vi "AprilTagFieldLayout_New2023.vi"() -> (3 "AprilTagFieldLayout":T1={"AprilTagMap"={}, "FieldLength"=0.0, "FieldWidth"=0.0, "OriginPosition "=enum."kBlueAllianceWallRightSide,", "OriginPose3d"={"Translation3d"={"X"=0.0, "Y"=0.0, "Z"=0.0}, "Rotation3d"={"Q_quaternion"={"R"=1.0, "V"=[0.0, 0.0, 0.0]}}}} {"OriginPose3d"."Translation3d"."Z" format="%14.3f"; "OriginPose3d"."Translation3d"."Y" format="%14.3f"; "OriginPose3d"."Translation3d"."X" format="%14.3f"})   [LabVIEW 2019, in "Trajectory_Library.lvlib"]
doc: "Define the FRC 2023 April Tag field layout.\n\nInputs:\n <none>\n\nOutputs:\n -- AprilTagFieldLayout -- AprilTagFieldLayout -- Data cluster containing field definition."
uses:
  Trajectory_Library.lvlib
  TypeDef/AprilTagFieldLayout.ctl
  TypeDef/AprilTag.ctl
  TypeDef/POSE3D.ctl
  TypeDef/TRANSLATION3D.ctl
  TypeDef/ROTATION3D.ctl
  TypeDef/QUATERNION.ctl
  Enum/AprilTagFieldLayoutOrignPosition_ENUM.ctl
  AprilTag_GetAll.vi
  Quaternion_Normalize.vi
  Quaternion_New_Default.vi
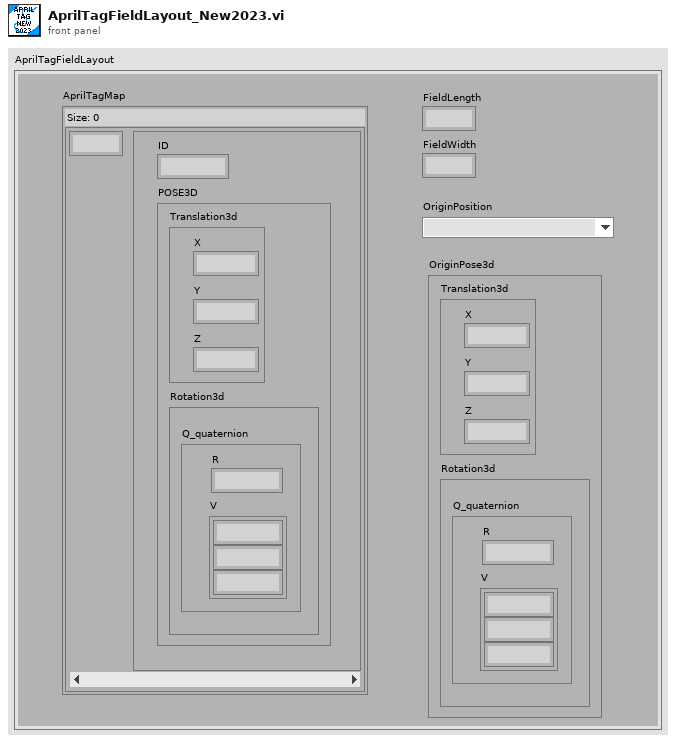
[diagram p1: front panel]
types:
  T1 = typedef "Trajectory_Library.lvlib/AprilTagFieldLayout.ctl" = cluster{"AprilTagMap":map{i32, T2}, "FieldLength":dbl, "FieldWidth":dbl, "OriginPosition ":T7, "OriginPose3d":T3}
  T2 = typedef "Trajectory_Library.lvlib/AprilTag.ctl" = cluster{"ID":i32, "POSE3D":T3}
  T3 = typedef "Trajectory_Library.lvlib/POSE3D.ctl" = cluster{"Translation3d":T4, "Rotation3d":T5}
  T4 = typedef "Trajectory_Library.lvlib/TRANSLATION3D.ctl" = cluster{"X":dbl, "Y":dbl, "Z":dbl}
  T5 = typedef "Trajectory_Library.lvlib/ROTATION3D.ctl" = cluster{"Q_quaternion":T6}
  T6 = typedef "Trajectory_Library.lvlib/QUATERNION.ctl" = cluster{"R":dbl, "V":dbl[]}
  T7 = typedef "Trajectory_Library.lvlib/AprilTagFieldLayoutOrignPosition_ENUM.ctl" = enum16{"kBlueAllianceWallRightSide,", "kRedAllianceWallRightSide,"}
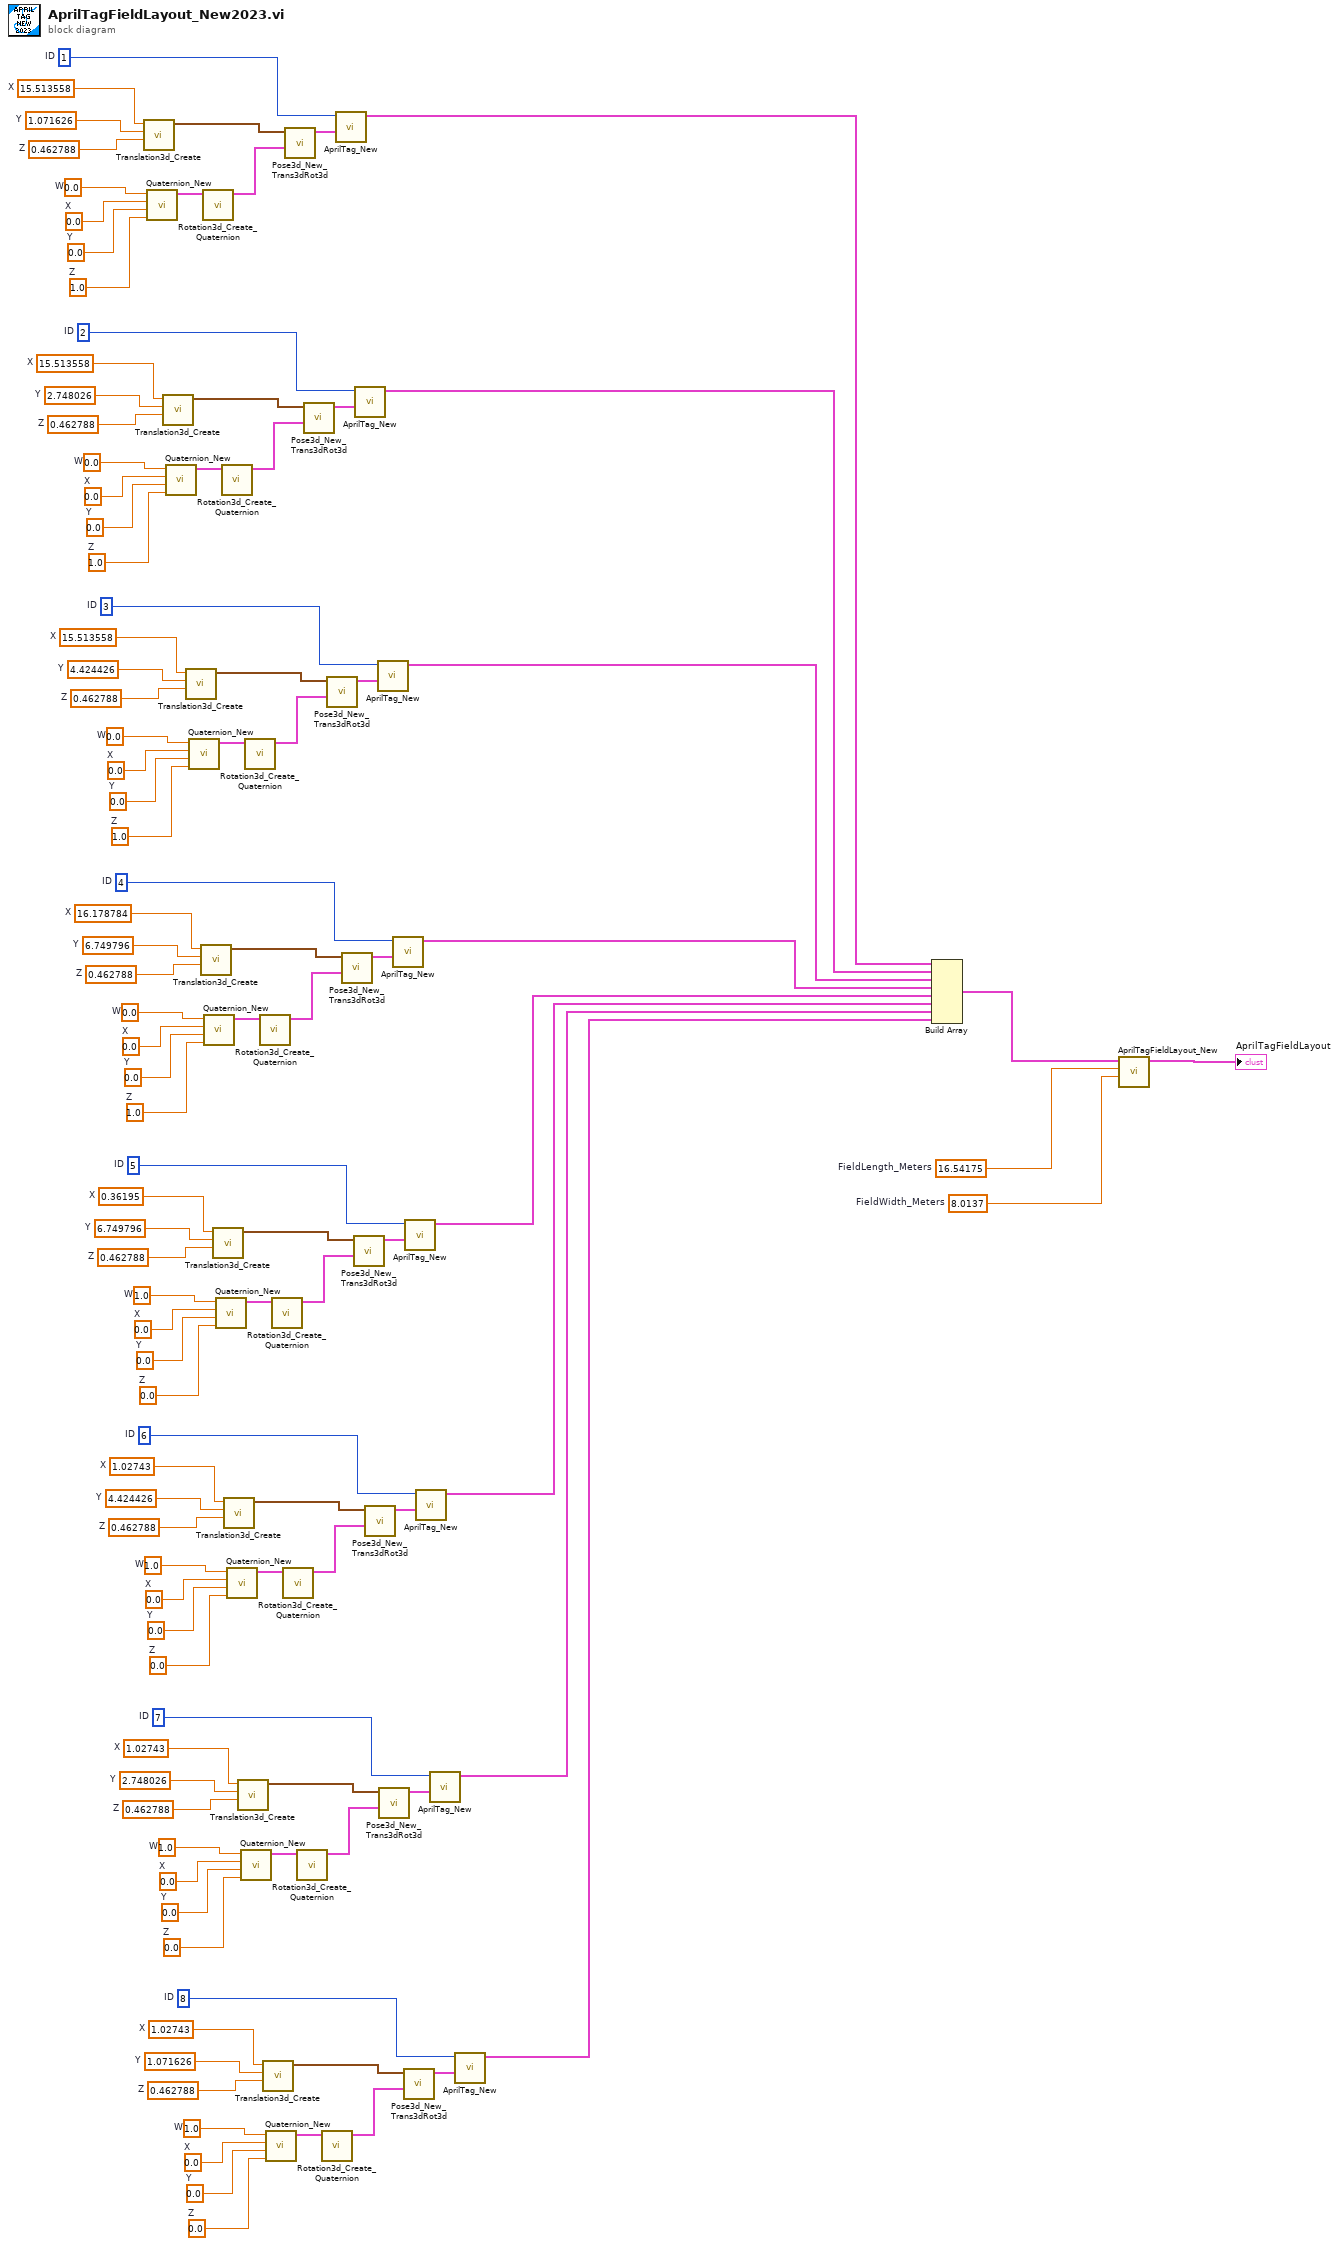
[diagram p0: block diagram]
diagram:
  w11 = 8  # ID
  w13 = 1.02743  # X
  w14 = 1.071626  # Y
  w15 = 0.462788  # Z
  w12 = 1.0  # W
  w16 = 0.0  # X
  w17 = 0.0  # Y
  w18 = 0.0  # Z
  w23 = 7  # ID
  w25 = 1.02743  # X
  w26 = 2.748026  # Y
  w27 = 0.462788  # Z
  w24 = 1.0  # W
  w28 = 0.0  # X
  w29 = 0.0  # Y
  w30 = 0.0  # Z
  w35 = 6  # ID
  w37 = 1.02743  # X
  w38 = 4.424426  # Y
  w39 = 0.462788  # Z
  w36 = 1.0  # W
  w40 = 0.0  # X
  w41 = 0.0  # Y
  w42 = 0.0  # Z
  w47 = 5  # ID
  w49 = 0.36195  # X
  w50 = 6.749796  # Y
  w51 = 0.462788  # Z
  w48 = 1.0  # W
  w52 = 0.0  # X
  w53 = 0.0  # Y
  w54 = 0.0  # Z
  w59 = 4  # ID
  w61 = 16.178784  # X
  w62 = 6.749796  # Y
  w63 = 0.462788  # Z
  w60 = 0.0  # W
  w64 = 0.0  # X
  w65 = 0.0  # Y
  w66 = 1.0  # Z
  w71 = 3  # ID
  w73 = 15.513558  # X
  w74 = 4.424426  # Y
  w75 = 0.462788  # Z
  w72 = 0.0  # W
  w76 = 0.0  # X
  w77 = 0.0  # Y
  w78 = 1.0  # Z
  w83 = 2  # ID
  w85 = 15.513558  # X
  w86 = 2.748026  # Y
  w87 = 0.462788  # Z
  w84 = 0.0  # W
  w88 = 0.0  # X
  w89 = 0.0  # Y
  w90 = 1.0  # Z
  w95 = 1  # ID
  w97 = 15.513558  # X
  w98 = 1.071626  # Y
  w99 = 0.462788  # Z
  w96 = 0.0  # W
  w100 = 0.0  # X
  w101 = 0.0  # Y
  w102 = 1.0  # Z
  w106 = 8.0137  # FieldWidth_Meters
  w107 = 16.54175  # FieldLength_Meters
  n1 = call "Translation3d_Create.vi"("Z"=w99, "Y"=w98, "X"=w97) -> ("TRANSLATION3D"=w105:T4)  [unwired: 8 in]
  n2 = call "Quaternion_New.vi"("Z"=w102, "Y"=w101, "X"=w100, "W"=w96) -> ("out Quaternion"=w103:T6)  [unwired: 7 in]
  n3 = call "Translation3d_Create.vi"("Z"=w87, "Y"=w86, "X"=w85) -> ("TRANSLATION3D"=w93:T4)  [unwired: 8 in]
  n4 = call "Quaternion_New.vi"("Z"=w90, "Y"=w89, "X"=w88, "W"=w84) -> ("out Quaternion"=w91:T6)  [unwired: 7 in]
  n5 = call "Translation3d_Create.vi"("Z"=w75, "Y"=w74, "X"=w73) -> ("TRANSLATION3D"=w81:T4)  [unwired: 8 in]
  n6 = call "Quaternion_New.vi"("Z"=w78, "Y"=w77, "X"=w76, "W"=w72) -> ("out Quaternion"=w79:T6)  [unwired: 7 in]
  n7 = call "Translation3d_Create.vi"("Z"=w63, "Y"=w62, "X"=w61) -> ("TRANSLATION3D"=w69:T4)  [unwired: 8 in]
  n8 = call "Rotation3d_Create_Quaternion.vi"("Quaternion"=w103) -> ("Rotation3d"=w104:T5)  [unwired: 10 in]
  n9 = call "Quaternion_New.vi"("Z"=w66, "Y"=w65, "X"=w64, "W"=w60) -> ("out Quaternion"=w67:T6)  [unwired: 7 in]
  n10 = call "Translation3d_Create.vi"("Z"=w51, "Y"=w50, "X"=w49) -> ("TRANSLATION3D"=w57:T4)  [unwired: 8 in]
  n11 = call "Quaternion_New.vi"("Z"=w54, "Y"=w53, "X"=w52, "W"=w48) -> ("out Quaternion"=w55:T6)  [unwired: 7 in]
  n12 = call "Rotation3d_Create_Quaternion.vi"("Quaternion"=w91) -> ("Rotation3d"=w92:T5)  [unwired: 10 in]
  n13 = call "Translation3d_Create.vi"("Z"=w39, "Y"=w38, "X"=w37) -> ("TRANSLATION3D"=w45:T4)  [unwired: 8 in]
  n14 = call "Quaternion_New.vi"("Z"=w42, "Y"=w41, "X"=w40, "W"=w36) -> ("out Quaternion"=w43:T6)  [unwired: 7 in]
  n15 = call "Translation3d_Create.vi"("Z"=w27, "Y"=w26, "X"=w25) -> ("TRANSLATION3D"=w33:T4)  [unwired: 8 in]
  n16 = call "Quaternion_New.vi"("Z"=w30, "Y"=w29, "X"=w28, "W"=w24) -> ("out Quaternion"=w31:T6)  [unwired: 7 in]
  n17 = call "Rotation3d_Create_Quaternion.vi"("Quaternion"=w79) -> ("Rotation3d"=w80:T5)  [unwired: 10 in]
  n18 = call "Rotation3d_Create_Quaternion.vi"("Quaternion"=w67) -> ("Rotation3d"=w68:T5)  [unwired: 10 in]
  n19 = call "Translation3d_Create.vi"("Z"=w15, "Y"=w14, "X"=w13) -> ("TRANSLATION3D"=w21:T4)  [unwired: 8 in]
  n20 = call "Quaternion_New.vi"("Z"=w18, "Y"=w17, "X"=w16, "W"=w12) -> ("out Quaternion"=w19:T6)  [unwired: 7 in]
  n21 = call "Rotation3d_Create_Quaternion.vi"("Quaternion"=w55) -> ("Rotation3d"=w56:T5)  [unwired: 10 in]
  n22 = call "Rotation3d_Create_Quaternion.vi"("Quaternion"=w43) -> ("Rotation3d"=w44:T5)  [unwired: 10 in]
  n23 = call "Pose3d_New_Trans3dRot3d.vi"("Rotation3d"=w104, "Translation3d"=w105) -> ("outPose3d"=w94:T3)  [unwired: 9 in]
  n24 = call "Rotation3d_Create_Quaternion.vi"("Quaternion"=w31) -> ("Rotation3d"=w32:T5)  [unwired: 10 in]
  n25 = call "Pose3d_New_Trans3dRot3d.vi"("Rotation3d"=w92, "Translation3d"=w93) -> ("outPose3d"=w82:T3)  [unwired: 9 in]
  n26 = call "Rotation3d_Create_Quaternion.vi"("Quaternion"=w19) -> ("Rotation3d"=w20:T5)  [unwired: 10 in]
  n27 = call "Pose3d_New_Trans3dRot3d.vi"("Rotation3d"=w80, "Translation3d"=w81) -> ("outPose3d"=w70:T3)  [unwired: 9 in]
  n28 = call "AprilTag_New.vi"("POSE3D"=w94, "ID"=w95) -> ("AprilTag"=w8:T2)  [unwired: 9 in]
  n29 = call "Pose3d_New_Trans3dRot3d.vi"("Rotation3d"=w68, "Translation3d"=w69) -> ("outPose3d"=w58:T3)  [unwired: 9 in]
  n30 = call "Pose3d_New_Trans3dRot3d.vi"("Rotation3d"=w56, "Translation3d"=w57) -> ("outPose3d"=w46:T3)  [unwired: 9 in]
  n31 = call "AprilTag_New.vi"("POSE3D"=w82, "ID"=w83) -> ("AprilTag"=w7:T2)  [unwired: 9 in]
  n32 = call "Pose3d_New_Trans3dRot3d.vi"("Rotation3d"=w44, "Translation3d"=w45) -> ("outPose3d"=w34:T3)  [unwired: 9 in]
  n33 = call "AprilTag_New.vi"("POSE3D"=w70, "ID"=w71) -> ("AprilTag"=w6:T2)  [unwired: 9 in]
  n34 = call "Pose3d_New_Trans3dRot3d.vi"("Rotation3d"=w32, "Translation3d"=w33) -> ("outPose3d"=w22:T3)  [unwired: 9 in]
  n35 = call "AprilTag_New.vi"("POSE3D"=w58, "ID"=w59) -> ("AprilTag"=w5:T2)  [unwired: 9 in]
  n36 = call "Pose3d_New_Trans3dRot3d.vi"("Rotation3d"=w20, "Translation3d"=w21) -> ("outPose3d"=w10:T3)  [unwired: 9 in]
  n37 = call "AprilTag_New.vi"("POSE3D"=w46, "ID"=w47) -> ("AprilTag"=w4:T2)  [unwired: 9 in]
  n38 = call "AprilTag_New.vi"("POSE3D"=w34, "ID"=w35) -> ("AprilTag"=w3:T2)  [unwired: 9 in]
  n39 = call "AprilTag_New.vi"("POSE3D"=w22, "ID"=w23) -> ("AprilTag"=w2:T2)  [unwired: 9 in]
  n40 = call "AprilTag_New.vi"("POSE3D"=w10, "ID"=w11) -> ("AprilTag"=w1:T2)  [unwired: 9 in]
  n41 = Build Array(w8, w7, w6, w5, w4, w3, w2, w1) -> (w9:T2[])
  n42 = call "AprilTagFieldLayout_New.vi"("FieldWidth_Meters"=w106, "FieldLength_Meters"=w107, "AprilTags"=w9) -> ("AprilTagFieldLayout"=→"AprilTagFieldLayout":T1)  [unwired: 8 in]
